vi "Run Process.vi"(6 "Parent VI":refnum<vi>, 8 "error in (no error)":errorcluster, 10 "Initial Parameters":cluster{"Initial Parameters":T1[]}[](array[cluster]), 11 "VI Ref In":refnum<vi>[](array[refnum])) -> (0 "error out":errorcluster, 3 "VI Ref In":refnum<vi>[](array[refnum]))   [LabVIEW 2015, in "FPGA Addon Engine.lvlib" / "Inline Async API.lvlib"]
uses:
  Inline Async API.lvlib
  Controls/Parameters Cluster.ctl
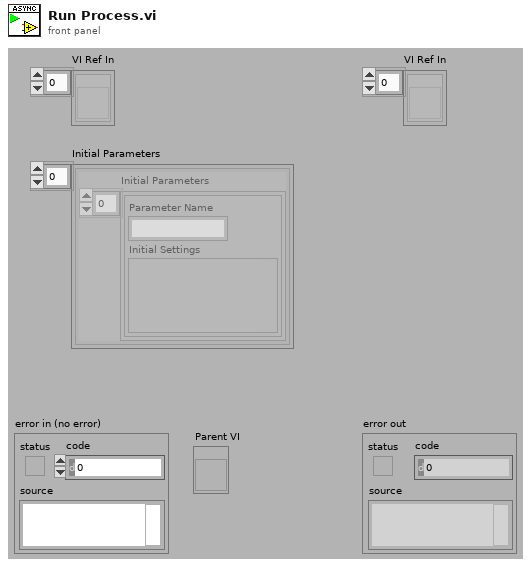
[diagram p1: front panel]
types:
  T1 = typedef "FPGA Addon Engine.lvlib/Inline Async API.lvlib/Parameters Cluster.ctl" = cluster{"Parameter Name":string, "Initial Settings":variant}
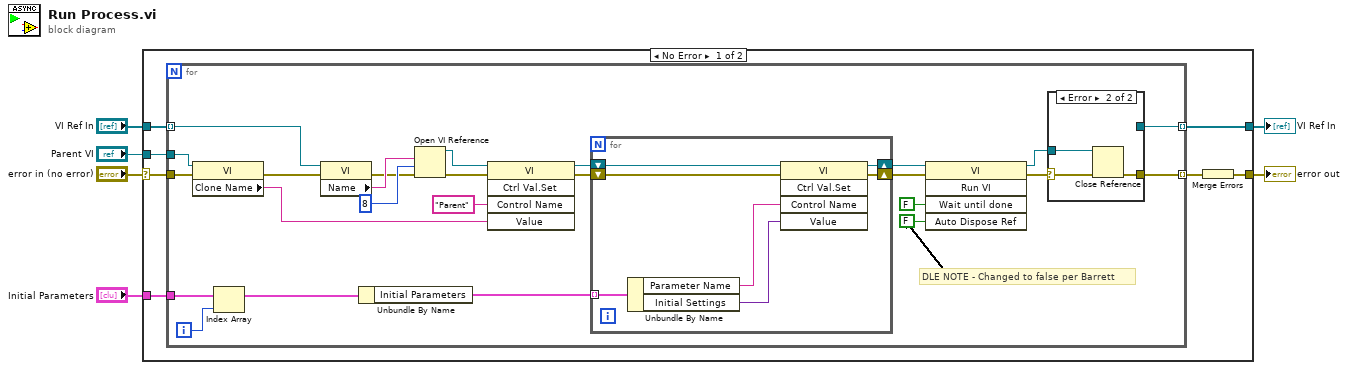
[diagram p0: block diagram]
diagram:
  n1 = case shown="No Error" "error in (no error)" {
    selector: "error in (no error)" -> [w10 w52]
    tunnel: [w7 w52] -> w6
    tunnel: "VI Ref In" -> [w12 w51]
    tunnel: [w11 w51] -> w4
    tunnel: "Initial Parameters" -> [w8 _]
    tunnel: "Parent VI" -> [w9 _]
    frame No Error {
      n2 = for {
        tunnel: [w38] -> w13 mode=indexing
        tunnel: w12 -> [w37] mode=indexing
        tunnel: [w36] -> w11 mode=indexing
        tunnel: w10 -> [w35]
        tunnel: w9 -> [w33]
        tunnel: w8 -> [w17]
        i -> [w14]
        # "DLE NOTE - Changed to false per Barrett"
        n3 = property class="VI"(reference=w33, error in=w35) -> (error out=w34:errorcluster, "Clone Name"=w32:string)  [unwired: 1 out]
        n4 = Index Array(array=w17, index=w14) -> (element=w15:cluster{"Initial Parameters":T1[]})
        n5 = property class="VI"(reference=w37, error in=w34) -> (error out=w23:errorcluster, "Name"=w31:string)  [unwired: 1 out]
        n6 = Unbundle By Name(w15) -> ("Initial Parameters"=w16:T1[])
        n7 = Open VI Reference(vi path=w31, options=8, error in (no error)=w23) -> (vi reference=w18:refnum<vi>, error out=w21:errorcluster)  [unwired: 3 out]
        n8 = invoke class="VI" method="Ctrl Val.Set"(reference=w18, error in=w21, "Control Name"="Parent", "Value"=w32) -> (reference out=w19:refnum<vi>, error out=w20:errorcluster)  [unwired: 1 in, 3 out]
        n9 = for {
          tunnel: w16 -> [w41] mode=indexing
          shift-right: [w44] -> w25
          shift-left: w19 -> [w42]
          shift-right: [w45] -> w26
          shift-left: w20 -> [w43]
          n10 = Unbundle By Name(w41) -> ("Parameter Name"=w40:string, "Initial Settings"=w39:variant)
          n11 = invoke class="VI" method="Ctrl Val.Set"(reference=w42, error in=w43, "Control Name"=w40, "Value"=w39) -> (reference out=w44:refnum<vi>, error out=w45:errorcluster)  [unwired: 1 in, 3 out]
        }
        n12 = invoke class="VI" method="Run VI"(reference=w25, error in=w26, "Wait until done"=FALSE ("Wait Until Done"), "Auto Dispose Ref"=FALSE ("Auto Dispose Reference")) -> (reference out=w27:refnum<vi>, error out=w28:errorcluster)  [unwired: 1 in, 3 out]
        n13 = case shown="Error" w28 {
          selector: w28 -> [w47 w50]
          tunnel: w27 -> [w46 w49]
          tunnel: [w47 w48] -> w38
          tunnel: [w46 _] -> w36
          frame No Error {
          }
          frame Error {
            n14 = Close Reference(reference=w49, error in (no error)=w50) -> (error out=w48:errorcluster)
          }
        }
      }
      n15 = Merge Errors(w13) -> (w7:errorcluster)
    }
    frame Error {
    }
  }
  "error out" <- w6
  "VI Ref In" <- w4
